vi "getStatus.vi"(8 "error in (no error)":errorcluster, 11 "Inst.Transport in":refnum<class "Inst.Transport.lvclass">) -> (0 "error out":errorcluster, 2 "Status":T1, 3 "Inst.Transport out":refnum<class "Inst.Transport.lvclass">)   [LabVIEW 2019, in "Inst.Transport.lvclass"]
uses:
  Inst.Transport.lvclass
  Typedefs/Inst.Transport.Status--Enum.ctl
  Typedefs/Inst.Transport.PublicCommands--Enum.ctl
  Typedefs/getStatus--Reply--Cluster.ctl
  b20095ea-c42e-4466-9ad9-90a293f3396f.vi
  b20095ea-c42e-4466-9ad9-90a293f3396f.vi/6e8856b0-d11e-429b-8e7f-ac706a745ea4.vi
  b20095ea-c42e-4466-9ad9-90a293f3396f.vi/aa3f4efd-e83e-4575-a096-eaa39c6fa10f.vi
  <vilib>/Utility/Data Type/Get Type Information.vi
  <vilib>/JDP Science/JSONtext/JSON text to Variant.vi
  <vilib>/JDP Science/JSONtext/LVClass Serializer/JSONtext LVClass Serializer.lvclass
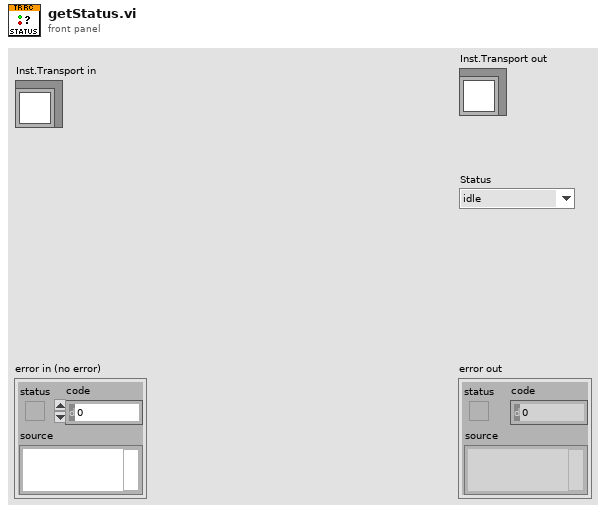
[diagram p1: front panel]
types:
  T1 = typedef "Inst.Transport.lvclass/Inst.Transport.Status--Enum.ctl" = enum16{"idle", "running"}
  T2 = typedef "Inst.Transport.lvclass/getStatus--Reply--Cluster.ctl" = cluster{"Status":T1}
  T3 = typedef "Inst.Transport.lvclass/Inst.Transport.PublicCommands--Enum.ctl" = enum16{"startTransport", "stopTransport", "getStatus", "setExptFolder", "setExptComments", "appendExptParam", "clearExptParam", "setExptParam", "setSweepConfig"}
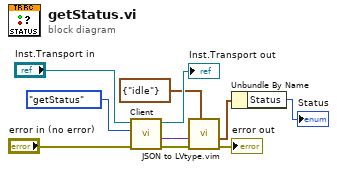
[diagram p0: block diagram]
diagram:
  n1 = call-dynamic "Client.vi"("error in (no error)"="error in (no error)", "Command in"=Inst.Transport.PublicCommands--Enum."getStatus" ("Commands"), "Instrument in"="Inst.Transport in") -> ("error out"=w2:errorcluster, "Data out"=w5:variant, "Instrument out"=→"Inst.Transport out":refnum<class "Inst.Transport.lvclass">)  [unwired: 5 in, 1 out]
  n2 = call "JSON to LVtype.vim"("type"=T2 {"Status"=enum."idle"} ("getStatus"), "error in (no error)"=w2, "JSON Data in"=w5) -> ("error out"=→"error out":errorcluster, "Data out"=w4:T2)  [unwired: 7 in]
  n3 = Unbundle By Name(w4) -> ("Status"=→"Status":T1)
